vi "GetFieldFromProtobufIndexGreeter_req_req_oneof.vi"(1 "protobuf index":i32) -> (0 "oneof field name":string)   [LabVIEW 2019, in "Generated_server.lvlib" / "Greeter_req_req_oneof.lvclass"]
uses:
  Greeter_req_req_oneof.lvclass
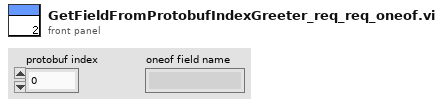
[diagram p1: front panel]
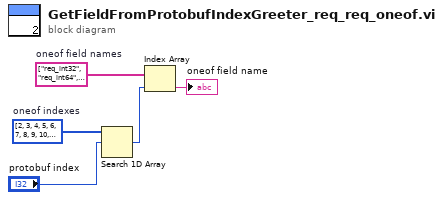
[diagram p0: block diagram]
diagram:
  w5 = string[] ["req_int32", "req_int64", "req_uint32", "req_uint64", "req_sint32", "req_sint64", "req_fixed32", "req_fixed64", "req_sfixed32", "req_sfixed64", "req_float", "req_double", "req_bool", "req_string", "req_bytes", "req_int32", "req_int64", "req_uint32", "req_uint64", "req_sint32", "req_sint64", "req_fixed32", "req_fixed64", "req_sfixed32", "req_sfixed64", "req_float", "req_double", "req_bool", "req_string", "req_bytes"]  # oneof field names
  w4 = i32[] [2, 3, 4, 5, 6, 7, 8, 9, 10, 11, 12, 13, 14, 15, 16, 2, 3, 4, 5, 6, 7, 8, 9, 10, 11, 12, 13, 14, 15, 16]  # oneof indexes
  n1 = Search 1D Array(1D array=w4, element="protobuf index") -> (index of element=w2:i32)  [unwired: 1 in]
  n2 = Index Array(array=w5, index=w2) -> (element=→"oneof field name":string)
